vi "Serial_Set(SCI_write).vi"(2 "baud rate (9600)":u32=115200 caption="보 전송속도(9600)", 3 "BAUD(9600)":string, 4 "Port":refnum<visa-resource-name>="COM4" caption="VISA 리소스 이름") -> (0 "Error Out":errorcluster caption="에러 출력", 1 "VISA out":refnum<visa-resource-name>)   [LabVIEW 2010]
uses:
  <vilib>/Instr/_visa.llb/VISA Flush IO Buffer Mask.ctl
  <vilib>/Instr/_visa.llb/VISA Configure Serial Port (Instr).vi
panel:
  out "Commend Count":u32
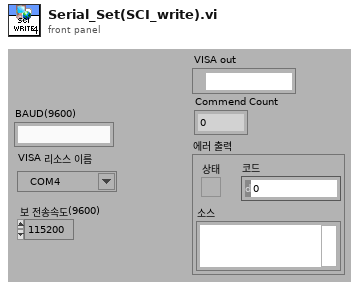
[diagram p1: front panel]
types:
  T1 = typedef "VISA Flush IO Buffer Mask.ctl" = u16
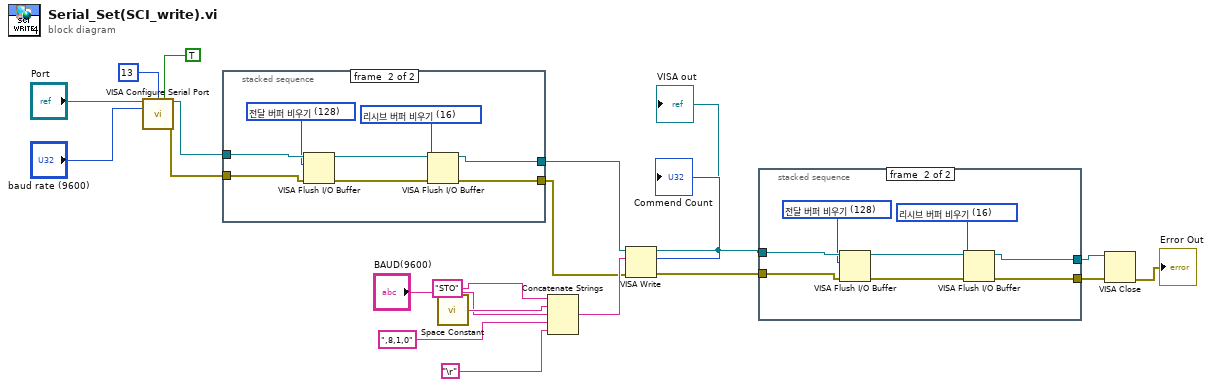
[diagram p0: block diagram]
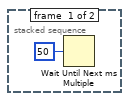
[diagram p2: hidden frame]
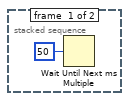
[diagram p3: hidden frame]
diagram:
  n1 = call-poly "VISA Configure Serial Port"("VISA resource name"="Port", "termination char\n(0xA = '\\n' = LF)"=i16 13 ("termination char\n(0xA = '\\n' = LF)"), "Enable Termination\nChar (T)"=TRUE ("Enable Termination\nChar (T)"), "baud rate (9600)"="baud rate (9600)") -> ("VISA resource name out"=w11:refnum<visa-resource-name>, "error out"=w10:errorcluster)  [unwired: 10 in]
  n2 = stacked-sequence {
    tunnel: w11 -> [_ w29]
    tunnel: w10 -> [_ w28]
    tunnel: [_ w24] -> w9
    tunnel: [_ w23] -> w8
    frame #0 {
      n3 = Wait Until Next ms Multiple(millisecond multiple=u32 50 ("ms 배수")) -> ()  [unwired: 1 out]
    }
    frame #1 {
      w22 = T1 16 items=["리시브 버퍼 비우기"=16, "전달 버퍼 디바이스에 쓰기"=32, "리시브 버퍼 비우기(I/O 없음)"=64, "전달 버퍼 비우기"=128] ("Mask")
      w27 = T1 128 items=["리시브 버퍼 비우기"=16, "전달 버퍼 디바이스에 쓰기"=32, "리시브 버퍼 비우기(I/O 없음)"=64, "전달 버퍼 비우기"=128] ("Mask")
      n4 = VISA Flush I/O Buffer(VISA resource name=w29, mask (16)=w27, error in (no error)=w28) -> (VISA resource name out=w26:refnum<visa-resource-name>, error out=w25:errorcluster)
      n5 = VISA Flush I/O Buffer(VISA resource name=w26, mask (16)=w22, error in (no error)=w25) -> (VISA resource name out=w24:refnum<visa-resource-name>, error out=w23:errorcluster)
    }
  }
  n6 = call <vilib>:"Space Constant.vi"() -> ("String"=w19:string)
  n7 = Concatenate Strings("STO", w19, "BAUD(9600)", ",8,1,0" ("문자열"), "\r") -> (w17:string)
  n8 = VISA Write(VISA resource name=w9, write buffer=w17, error in (no error)=w8) -> (VISA resource name out=w5:refnum<visa-resource-name>, return count=→"Commend Count":u32, error out=w4:errorcluster)
  "VISA out" <- w5
  n9 = stacked-sequence {
    tunnel: w5 -> [_ w38]
    tunnel: w4 -> [_ w37]
    tunnel: [_ w33] -> w6
    tunnel: [_ w32] -> w7
    frame #0 {
      n10 = Wait Until Next ms Multiple(millisecond multiple=u32 50 ("ms 배수")) -> ()  [unwired: 1 out]
    }
    frame #1 {
      w31 = T1 16 items=["리시브 버퍼 비우기"=16, "전달 버퍼 디바이스에 쓰기"=32, "리시브 버퍼 비우기(I/O 없음)"=64, "전달 버퍼 비우기"=128] ("Mask")
      w36 = T1 128 items=["리시브 버퍼 비우기"=16, "전달 버퍼 디바이스에 쓰기"=32, "리시브 버퍼 비우기(I/O 없음)"=64, "전달 버퍼 비우기"=128] ("Mask")
      n11 = VISA Flush I/O Buffer(VISA resource name=w38, mask (16)=w36, error in (no error)=w37) -> (VISA resource name out=w35:refnum<visa-resource-name>, error out=w34:errorcluster)
      n12 = VISA Flush I/O Buffer(VISA resource name=w35, mask (16)=w31, error in (no error)=w34) -> (VISA resource name out=w33:refnum<visa-resource-name>, error out=w32:errorcluster)
    }
  }
  n13 = VISA Close(VISA resource name=w6, error in (no error)=w7) -> (error out=→"Error Out":errorcluster)
